vi "Begin.vi"() -> (0 "error out":errorcluster)   [LabVIEW 2011]
doc: "Called before other user functions, this VI is expected to open initial I/O refnums, load in file data, and do all program initialization. Notice that the <B>error out</B> terminal is simply used for data flow. Wiring it to other structures or subVIs ensures that this VI runs first."
uses:
  <vilib>/Rock Robotics/SystemInterfaces/DIO/FPGA_DIOPWMChannel.ctl
  <vilib>/Rock Robotics/WPI/Joystick/WPI_JoystickDeviceEnum.ctl
  <vilib>/Rock Robotics/SystemInterfaces/Typedef/FPGA_TypedefDigitalModule.ctl
  <vilib>/Rock Robotics/SystemInterfaces/DIO/FPGA_DIORelayChannel.ctl
  <vilib>/Rock Robotics/WPI/MotorControl/WPI_MotorControlOpen Victor.vi
  <vilib>/Rock Robotics/WPI/MotorControl/WPI_MotorControlOpen Jaguar.vi
  Robot Global Data.vi
panel:
  out "Global: Auton Files":string[](array[string])
  out "Global: Auton Array":dbl[][](array[numeric])
  out "Global: Current Auton File":string
  out "Global: Number of Auton Files":i64
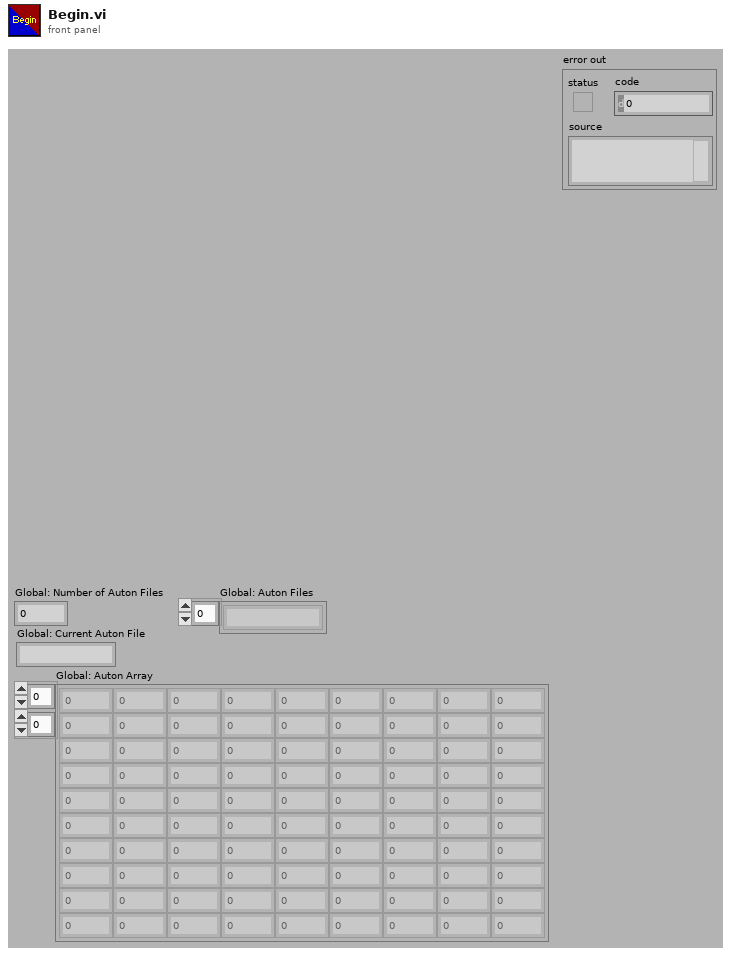
[diagram p1: front panel]
types:
  T1 = typedef "FPGA_DIORelayChannel.ctl" = enum8{"Relay 1", "Relay 2", "Relay 3", "Relay 4", "Relay 5", "Relay 6", "Relay 7", "Relay 8", "Invalid"}
  T2 = typedef "FPGA_TypedefDigitalModule.ctl" = enum16{"Digital Module 1", "Digital Module 2"}
  T3 = typedef "WPI_JoystickDeviceEnum.ctl" = enum16{"USB 1", "USB 2", "USB 3", "USB 4", "Kinect 1", "Kinect 2"}
  T4 = typedef "FPGA_DIOPWMChannel.ctl" = enum8{"PWM 1", "PWM 2", "PWM 3", "PWM 4", "PWM 5", "PWM 6", "PWM 7", "PWM 8", "PWM 9", "PWM 10", "Invalid"}
  T5 = typedef "WPI_CameraImageSize.ctl" = enum16{"640x480", "320x240", "160x120"}
  T6 = cluster{"fps":i32, "compression":i32, "Image Size":T5}
  T7 = typedef "WPI_CameraWhite Balance Values.ctl" = enum16{"Auto", "Fixed indoor", "Fixed outdoor 1", "Fixed outdoor 2", "Fixed fluorescent 1", "Fixed fluorescent 2", "Hold current"}
  T8 = typedef "WPI_ServoDeviceRef.ctl" = cluster{"DeviceStatus":errorcluster, "Digital Module":T2, "PWM Channel":T4, "DeadBand":T9}
  T9 = typedef "WPI_PWMDeadband.ctl" = cluster{"Name":string, "maxPositivePwm":i32, "minPositivePwm":i32, "centerPwm":i32, "maxNegativePwm":i32, "minNegativePwm":i32, "angularRange":u16}
  T10 = typedef "WPI_CameraDevRef.ctl" = cluster{"Camera Address":string, "CameraStatus":errorcluster, "Acquire Image Notifier":refnum<notifier>}
  T11 = typedef "WPI_MotorControlDeviceRef.ctl" = cluster{"DeviceStatus":errorcluster, "Type":enum16{"PWM", "CAN"}, "PWM":cluster{"Digital Module":T2, "PWM Channel":T4, "DeadBand":T9}, "CAN":cluster{"Device Number":u8, "Control Mode":T12, "Semaphore":T13, "Max Vout":dbl}, "Invert":bool, "TransformRef":T14, "InvTransformRef":T14}
  T12 = typedef "WPI_CANJaguar_ControlMode.ctl" = enum8{"Percent VBus", "Current", "Speed", "Position", "Voltage"}
  T13 = typedef "Semaphore RefNum" = refnum<k1>
  T14 = typedef "WPI_PWMTransform_ConPane.ctl" = refnum<vi>
  T15 = typedef "WPI_CameraExposure Values.ctl" = enum16{"Auto", "Flicker-free 50 Hz", "Flicker-free 60 Hz", "Hold current"}
  T16 = typedef "WPI_RelayDevRef.ctl" = cluster{"DevStatus":errorcluster, "Relay Channel":T1, "Digital Module":T2, "Relay Direction":T17}
  T17 = typedef "WPI_RelayDirection.ctl" = enum16{"Both directions", "Forward only", "Reverse only"}
  T18 = typedef "WPI_JoystickDevRef.ctl" = cluster{"Device":T3}
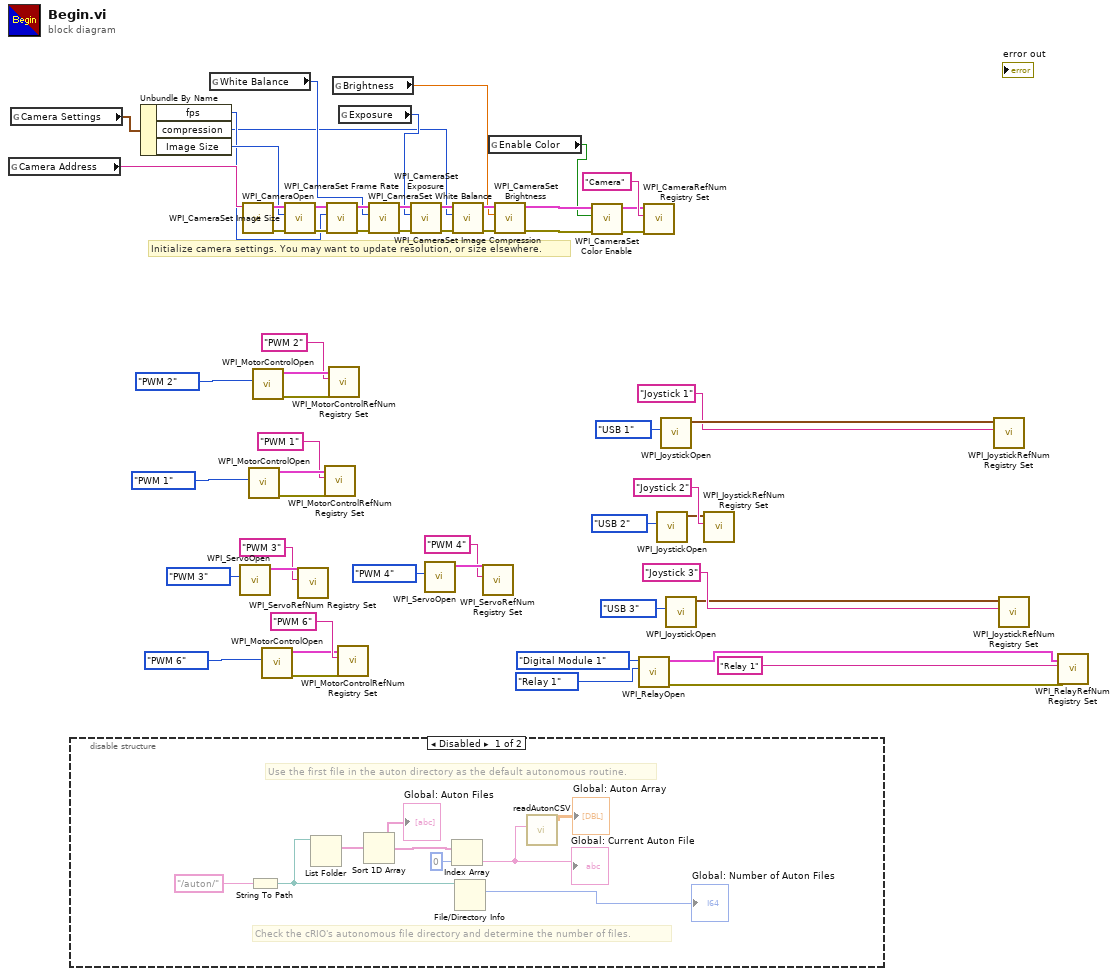
[diagram p0: block diagram]
diagram:
  # "Initialize camera settings. You may want to update resolution, or size elsewhere."
  n1 = global read "Robot Global Data.vi" "Camera Address"() -> (w45:string)
  n2 = global read "Robot Global Data.vi" "Camera Settings"() -> (w12:T6)
  n3 = disable-structure shown="Disabled" {
    frame Disabled {
      # "Check the cRIO's autonomous file directory and determine the number of files."
      # "Use the first file in the auton directory as the default autonomous routine."
      n4 = String To Path(string="/auton/") -> (path=w65:path)
      n5 = List Folder(path=w65) -> (filenames=w64:string[])  [unwired: 1 in, 5 out]
      n6 = Sort 1D Array(array=w64) -> (sorted array=w62:string[])
      "Global: Auton Files" <- w62
      n7 = Index Array(array=w62, index=0) -> (element=w60:string)
      "Global: Current Auton File" <- w60
      n8 = File/Directory Info(path=w65) -> (size=→"Global: Number of Auton Files":i64)  [unwired: 1 in, 6 out]
      n9 = call "readAutonCSV.vi"("AutonFile"=w60) -> ("AutonArray"=→"Global: Auton Array":dbl[][])  [unwired: 7 in]
    }
    frame Enabled {
    }
  }
  n10 = Unbundle By Name(w12) -> ("fps"=w10:i32, "compression"=w7:i32, "Image Size"=w11:T5)
  n11 = global read "Robot Global Data.vi" "White Balance"() -> (w9:T7)
  n12 = call <vilib>:"WPI_ServoOpen.vi"("PWM Channel"=FPGA_DIOPWMChannel."PWM 3") -> ("ServoDeviceRef"=w31:T8)  [unwired: 9 in, 1 out]
  n13 = call <vilib>:"WPI_CameraOpen.vi"("Camera Address"=w45) -> ("error out"=w51:errorcluster, "CameraDevRef"=w52:T10)  [unwired: 1 in, 8 out]
  n14 = call-poly <vilib>:"WPI_MotorControlOpen.vi"("PWM Channel"=FPGA_DIOPWMChannel."PWM 1") -> ("error out"=w37:errorcluster, "MotorControlDeviceRef"=w40:T11)  [unwired: 9 in]
  n15 = call-poly <vilib>:"WPI_MotorControlOpen.vi"("PWM Channel"=FPGA_DIOPWMChannel."PWM 2") -> ("error out"=w38:errorcluster, "MotorControlDeviceRef"=w43:T11)  [unwired: 9 in]
  n16 = call-poly <vilib>:"WPI_MotorControlOpen.vi"("PWM Channel"=FPGA_DIOPWMChannel."PWM 6") -> ("error out"=w26:errorcluster, "MotorControlDeviceRef"=w24:T11)  [unwired: 9 in]
  n17 = call <vilib>:"WPI_CameraSet Image Size.vi"("error in (no error)"=w51, "Image Size"=w11, "CameraDevRef"=w52) -> ("error out"=w50:errorcluster, "CameraDevRef Out"=w53:T10)  [unwired: 7 out]
  n18 = call <vilib>:"WPI_ServoRefNum Registry Set.vi"("refnum name"="PWM 3", "ServoDeviceRef"=w31) -> ()  [unwired: 8 in, 2 out]
  n19 = call <vilib>:"WPI_MotorControlRefNum Registry Set.vi"("error in (no error)"=w37, "refnum name"="PWM 1", "MotorControlDevRef"=w40) -> ()  [unwired: 7 in, 2 out]
  n20 = call <vilib>:"WPI_CameraSet Frame Rate.vi"("error in (no error)"=w50, "Frame Rate (fps)"=w10, "CameraDevRef"=w53) -> ("error out"=w49:errorcluster, "CameraDevRef Out"=w55:T10)  [unwired: 7 out]
  n21 = call <vilib>:"WPI_MotorControlRefNum Registry Set.vi"("error in (no error)"=w38, "refnum name"="PWM 2", "MotorControlDevRef"=w43) -> ()  [unwired: 7 in, 2 out]
  n22 = global read "Robot Global Data.vi" "Brightness"() -> (w6:dbl)
  n23 = call <vilib>:"WPI_MotorControlRefNum Registry Set.vi"("error in (no error)"=w26, "refnum name"="PWM 6", "MotorControlDevRef"=w24) -> ()  [unwired: 7 in, 2 out]
  n24 = global read "Robot Global Data.vi" "Exposure"() -> (w8:T15)
  n25 = call <vilib>:"WPI_CameraSet White Balance.vi"("error in (no error)"=w49, "White Balance"=w9, "CameraDevRef"=w55) -> ("error out"=w48:errorcluster, "CameraDevRef Out"=w54:T10)  [unwired: 7 out]
  n26 = call <vilib>:"WPI_CameraSet Exposure.vi"("error in (no error)"=w48, "Exposure"=w8, "CameraDevRef"=w54) -> ("error out"=w47:errorcluster, "CameraDevRef Out"=w57:T10)  [unwired: 7 out]
  n27 = call <vilib>:"WPI_ServoOpen.vi"("PWM Channel"=FPGA_DIOPWMChannel."PWM 4") -> ("ServoDeviceRef"=w29:T8)  [unwired: 9 in, 1 out]
  n28 = call <vilib>:"WPI_CameraSet Image Compression.vi"("error in (no error)"=w47, "Compression"=w7, "CameraDevRef"=w57) -> ("error out"=w46:errorcluster, "CameraDevRef Out"=w56:T10)  [unwired: 7 out]
  n29 = call <vilib>:"WPI_ServoRefNum Registry Set.vi"("refnum name"="PWM 4", "ServoDeviceRef"=w29) -> ()  [unwired: 8 in, 2 out]
  n30 = global read "Robot Global Data.vi" "Enable Color"() -> (w1:bool)
  n31 = call <vilib>:"WPI_CameraSet Brightness.vi"("error in (no error)"=w46, "Brightness"=w6, "CameraDevRef"=w56) -> ("error out"=w4:errorcluster, "CameraDevRef Out"=w5:T10)  [unwired: 7 out]
  n32 = call <vilib>:"WPI_CameraSet Color Enable.vi"("error in (no error)"=w4, "Color Enabled"=w1, "CameraDevRef"=w5) -> ("error out"=w2:errorcluster, "CameraDevRef Out"=w3:T10)  [unwired: 7 in]
  n33 = call <vilib>:"WPI_RelayOpen.vi"("Relay Channel"=FPGA_DIORelayChannel."Relay 1", "Digital Module (Module 1)"=FPGA_TypedefDigitalModule."Digital Module 1") -> ("error out"=w15:errorcluster, "RelayDevRef"=w16:T16)  [unwired: 8 in]
  n34 = call <vilib>:"WPI_CameraRefNum Registry Set.vi"("error in (no error)"=w2, "refnum name"="Camera", "CameraDevRef"=w3) -> ()  [unwired: 9 out]
  n35 = call <vilib>:"WPI_JoystickOpen.vi"("JoystickDevice"=WPI_JoystickDeviceEnum."USB 2") -> ("JoystickDevRef"=w33:T18)  [unwired: 10 in]
  n36 = call <vilib>:"WPI_JoystickOpen.vi"("JoystickDevice"=WPI_JoystickDeviceEnum."USB 1") -> ("JoystickDevRef"=w36:T18)  [unwired: 10 in]
  n37 = call <vilib>:"WPI_JoystickOpen.vi"("JoystickDevice"=WPI_JoystickDeviceEnum."USB 3") -> ("JoystickDevRef"=w21:T18)  [unwired: 10 in]
  n38 = call <vilib>:"WPI_JoystickRefNum Registry Set.vi"("refnum name"="Joystick 2", "JoystickDevRef"=w33) -> ()  [unwired: 8 in, 2 out]
  n39 = call <vilib>:"WPI_JoystickRefNum Registry Set.vi"("refnum name"="Joystick 1", "JoystickDevRef"=w36) -> ()  [unwired: 8 in, 2 out]
  n40 = call <vilib>:"WPI_JoystickRefNum Registry Set.vi"("refnum name"="Joystick 3", "JoystickDevRef"=w21) -> ()  [unwired: 8 in, 2 out]
  n41 = call <vilib>:"WPI_RelayRefNum Registry Set.vi"("error in (no error)"=w15, "refnum name"="Relay 1", "RelayDevRef"=w16) -> ()  [unwired: 7 in, 2 out]
